vi "test_table_creation.vi"(8 "error in (no error)":errorcluster) -> (0 "error out":errorcluster, 3 "trimmed string":string)   [LabVIEW 2020]
uses:
  75441b51-3bf2-4981-8bbc-1672bc4a7a0b.vi
  75441b51-3bf2-4981-8bbc-1672bc4a7a0b.vi/4178f046-9af6-4db4-9405-99552d650b27.vi
  75441b51-3bf2-4981-8bbc-1672bc4a7a0b.vi/504846f3-46c1-483c-ab2c-e4b1da560c38.vi
  toml/write_subtable_key_string.vi
  <vilib>/addons/_JKI Toolkits/Caraya/classes/Assert/Assert True.vi
  <vilib>/addons/_JKI Toolkits/Caraya/classes/Assert/Assert False.vi
  <vilib>/addons/_JKI Toolkits/Caraya/classes/Assert/Assert Not Error.vi
  toml/toml.lvclass
  <vilib>/addons/_JKI Toolkits/Caraya/classes/Assert/Assert.lvclass
  <vilib>/addons/_JKI Toolkits/Caraya/classes/Test/Test.lvclass
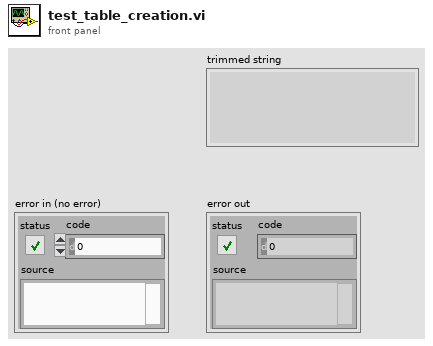
[diagram p1: front panel]
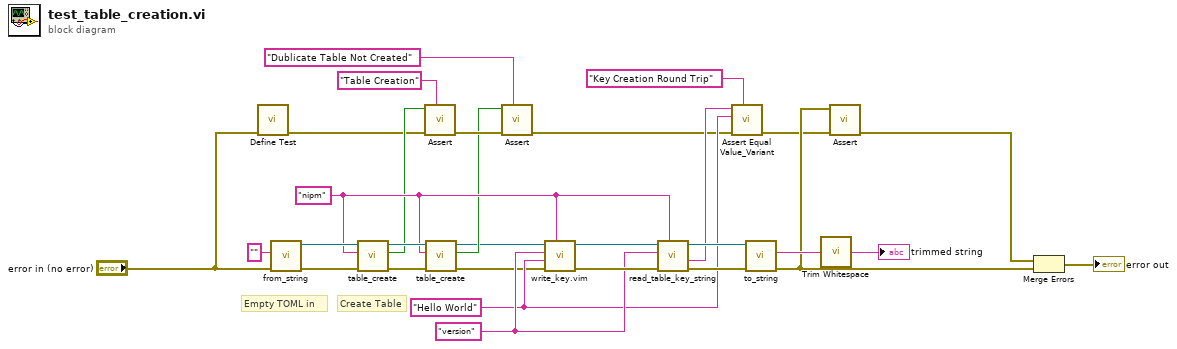
[diagram p0: block diagram]
diagram:
  w17 = "Hello World" ("value")
  w18 = "version" ("key")
  w14 = "nipm" ("table_name")
  # "Create Table"
  # "Empty TOML in"
  n1 = call <vilib>:"Define Test.vi"("error in (no error)"="error in (no error)") -> ("error out"=w11:errorcluster)  [unwired: 10 in]
  n2 = call "from_string.vi"("error in (no error)"="error in (no error)", "toml"="") -> ("error out"=w19:errorcluster, "toml out"=w20:refnum<class "toml.lvclass">)  [unwired: 8 in]
  n3 = call "table_create.vi"("error in (no error)"=w19, "table name"=w14, "toml in"=w20) -> ("error out"=w7:errorcluster, "table created"=w12:bool, "toml out"=w15:refnum<class "toml.lvclass">)  [unwired: 6 in]
  n4 = call-poly <vilib>:"Assert.vi"("Label"="Table Creation", "error in (no error)"=w11, "True?"=w12) -> ("error out"=w10:errorcluster)  [unwired: 8 in]
  n5 = call "table_create.vi"("error in (no error)"=w7, "table name"=w14, "toml in"=w15) -> ("error out"=w5:errorcluster, "table created"=w8:bool, "toml out"=w6:refnum<class "toml.lvclass">)  [unwired: 6 in]
  n6 = call-poly <vilib>:"Assert.vi"("Label"="Dublicate Table Not Created", "error in (no error)"=w10, "False?"=w8) -> ("error out"=w4:errorcluster)  [unwired: 8 in]
  n7 = call "write_key.vim"("table"=w14, "error in (no error)"=w5, "value"=w17, "key"=w18, "toml in"=w6) -> ("error out"=w30:errorcluster, "toml out"=w28:refnum<class "toml.lvclass">)  [unwired: 5 in]
  n8 = call "read_table_key_string.vi"("table"=w14, "error in (no error)"=w30, "key"=w18, "toml in"=w28) -> ("error out"=w29:errorcluster, "value"=w26:string, "toml out"=w27:refnum<class "toml.lvclass">)  [unwired: 4 in, 1 out]
  n9 = call <vilib>:"Assert Equal Value_Variant.vi"("Label"="Key Creation Round Trip", "error in (no error)"=w4, "Y"=w17, "X"=w26) -> ("error out"=w2:errorcluster)  [unwired: 7 in]
  n10 = call "to_string.vi"("error in (no error)"=w29, "toml in"=w27) -> ("error out"=w3:errorcluster, "toml_string"=w22:string)  [unwired: 8 in]
  n11 = call <vilib>:"Trim Whitespace.vi"("string"=w22) -> ("trimmed string"=→"trimmed string":string)  [unwired: 1 in]
  n12 = call-poly <vilib>:"Assert.vi"("error in (no error)"=w2, "Not Error?"=w3) -> ("error out"=w1:errorcluster)  [unwired: 9 in]
  n13 = Merge Errors(w1, w3) -> (→"error out":errorcluster)
